vi "DataFileCreator2.vi"(10 "ProjectName":string="PrWave", 11 "Folder path input":path=path "C:/Users/Lab/Desktop/Data/DataBristol") -> (2 "NewFileCreated":string, 3 "NewFilePath":path)   [LabVIEW 2016]
doc: "Given an input Folder path this VI creates the next data file in the format \n2017-09-17ProjectName#001\nIt only checks the latest file in the folder to decide if a sequence with today's date already exists.\nIf the file sequence has not been started, it creates one begining with #001\nIf it happens that it tries to create a file that already exists, a dialog pops up\nasking for a new name."
panel:
  out "File time stamps sorted by time":timestamp[](array[timestamp])
  out "Files in Folder sorted by time":path[](array[path])
  out "FileTypeExists?":bool
  out "date string":string
  out "YearNow":string
  out "DayNow":string
  out "MonthNow":string
  out "DayParsed":string
  out "MonthParsed":string
  out "YearParsed":string
  out "newest existing file":string
  # "Given an input Folder path this VI creates the next data file in the format \n2017-09-17ProjectName#001\nIt only checks the latest file in the folder to decide if \na sequence with today's date already exists.\nIf the file sequence has not been started, it creates one begining with #001\nIf it happens that it tries to create a file that already exists, a dialog pops up\nasking for a new name."
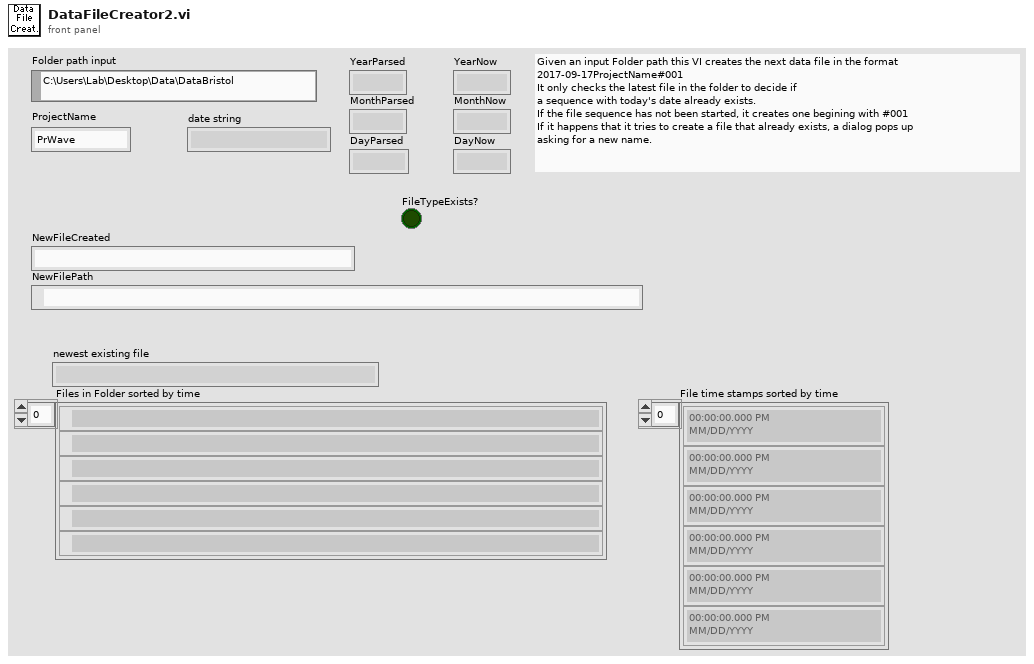
[diagram p1: front panel]
types:
  T1 = enum16{"open", "replace", "create", "open or create", "replace or create", "replace or create with confirmation"}
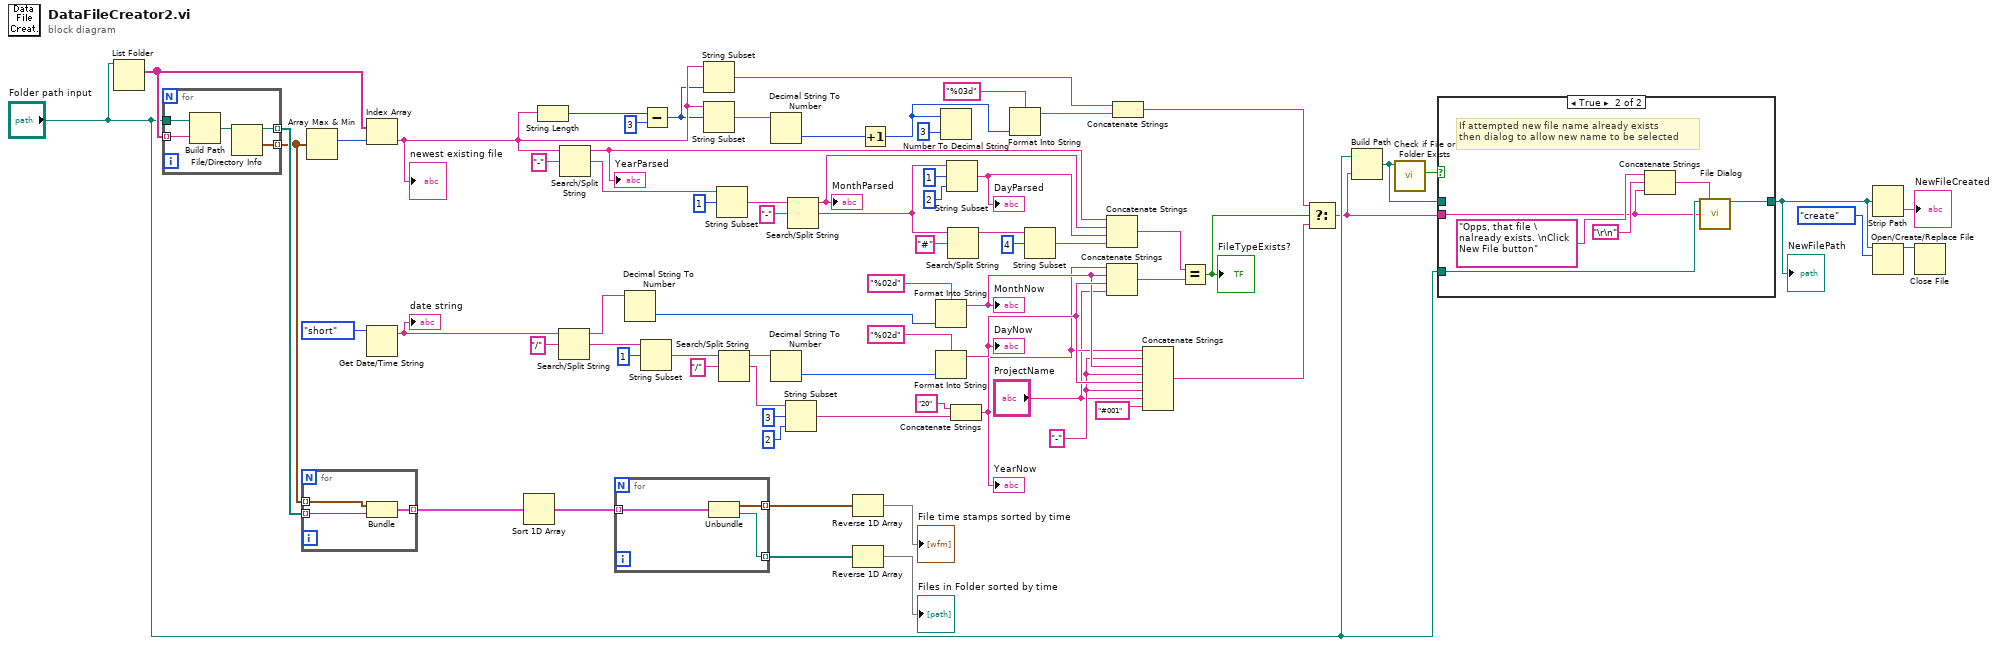
[diagram p0: block diagram]
diagram:
  w37 = "-" ("string")
  n1 = List Folder(path="Folder path input") -> (filenames=w51:string[])  [unwired: 3 in, 3 out]
  n2 = for {
    tunnel: w51 -> [w78] mode=indexing
    tunnel: [w76] -> w8 mode=indexing
    tunnel: [w75] -> w7 mode=indexing
    tunnel: "Folder path input" -> [w74]
    n3 = Build Path(base path=w74, name or relative path=w78) -> (appended path=w77:path)
    n4 = File/Directory Info(path=w77) -> (path out=w76:path, last mod=w75:timestamp)  [unwired: 1 in, 5 out]
  }
  n5 = for {
    tunnel: w7 -> [w81] mode=indexing
    tunnel: w8 -> [w80] mode=indexing
    tunnel: [w79] -> w14 mode=indexing
    n6 = Bundle("last mod"=w81, "path out"=w80) -> (w79:cluster{"last mod":timestamp, "path out":path})  [unwired: 1 in]
  }
  n7 = Array Max & Min(array=w7) -> (max index (indices)=w52:i32)  [unwired: 3 out]
  n8 = Index Array(array=w51, index=w52) -> (element=w42:string)
  "newest existing file" <- w42
  n9 = Get Date/Time String(date format (0)=enum16{"short", "long", "abbreviated"}."short") -> (date string=w55:string)  [unwired: 2 in, 1 out]
  "date string" <- w55
  n10 = Sort 1D Array(array=w14) -> (sorted array=w13:cluster{"last mod":timestamp, "path out":path}[])
  n11 = String Length(string=w42) -> (length=w32:i32)
  n12 = Search/Split String(string=w55, search string/char (-)="/") -> (substring before match=w47:string, match + rest of string=w63:string)  [unwired: 1 in, 1 out]
  n13 = Search/Split String(string=w42, search string/char (-)="-") -> (substring before match=w41:string, match + rest of string=w70:string)  [unwired: 1 in, 1 out]
  "YearParsed" <- w41
  n14 = for {
    tunnel: w13 -> [w84] mode=indexing
    tunnel: [w83] -> w11 mode=indexing
    tunnel: [w82] -> w12 mode=indexing
    n15 = Unbundle(w84) -> ("last mod"=w82:timestamp, "path out"=w83:path)
  }
  n16 = Decimal String To Number(string=w47) -> (number=w46:i32)  [unwired: 2 in, 1 out]
  n17 = String Subset(string=w63, offset (0)=1) -> (substring=w62:string)  [unwired: 1 in]
  n18 = Subtract(x=w32, y=3) -> (x-y=w30:i32)
  n19 = String Subset(string=w42, length (rest)=w30) -> (substring=w24:string)  [unwired: 1 in]
  n20 = String Subset(string=w42, offset (0)=w30) -> (substring=w29:string)  [unwired: 1 in]
  n21 = String Subset(string=w70, offset (0)=1) -> (substring=w69:string)  [unwired: 1 in]
  n22 = Search/Split String(string=w62, search string/char (-)="/") -> (substring before match=w43:string, match + rest of string=w60:string)  [unwired: 1 in, 1 out]
  n23 = Decimal String To Number(string=w29) -> (number=w28:i32)  [unwired: 2 in, 1 out]
  n24 = Decimal String To Number(string=w43) -> (number=w44:i32)  [unwired: 2 in, 1 out]
  n25 = String Subset(string=w60, offset (0)=3, length (rest)=2 ("y")) -> (substring=w57:string)
  n26 = Search/Split String(string=w69, search string/char (-)="-") -> (substring before match=w54:string, match + rest of string=w4:string)  [unwired: 1 in, 1 out]
  "MonthParsed" <- w54
  n27 = Reverse 1D Array(array=w12) -> (reversed array=→"File time stamps sorted by time":timestamp[])
  n28 = Reverse 1D Array(array=w11) -> (reversed array=→"Files in Folder sorted by time":path[])
  n29 = Increment(x=w28) -> (x+1=w26:i32)
  n30 = Format Into String(format string="%02d", w46) -> (resulting string=w39:string)  [unwired: 2 in, 1 out]
  "MonthNow" <- w39
  n31 = Format Into String(format string="%02d", w44) -> (resulting string=w40:string)  [unwired: 2 in, 1 out]
  "DayNow" <- w40
  n32 = Number To Decimal String(number=w26, width (-)=i16 3) -> ()  [unwired: 1 out]
  n33 = String Subset(string=w4, offset (0)=1, length (rest)=2 ("y")) -> (substring=w53:string)
  "DayParsed" <- w53
  n34 = Search/Split String(string=w4, search string/char (-)="#") -> (substring before match=w3:string)  [unwired: 1 in, 2 out]
  n35 = Concatenate Strings("20" ("string"), w57) -> (w38:string)
  "YearNow" <- w38
  n36 = Format Into String(format string="%03d", w26) -> (resulting string=w23:string)  [unwired: 2 in, 1 out]
  n37 = String Subset(string=w3, offset (0)=4) -> (substring=w2:string)  [unwired: 1 in]
  n38 = Concatenate Strings(w41, w54, w53, w2) -> (w50:string)
  n39 = Concatenate Strings(w38, w39, w40, "ProjectName") -> (w49:string)
  n40 = Concatenate Strings(w24, w23) -> (w34:string)
  n41 = Concatenate Strings(w38, w37, w39, w37, w40, w37, "ProjectName", "#001" ("string")) -> (w33:string)
  n42 = Equal?(x=w50, y=w49) -> (x = y?=w35:bool)
  "FileTypeExists?" <- w35
  n43 = Select(t=w34, s=w35, f=w33) -> (s? t:f=w17:string)
  n44 = Build Path(base path="Folder path input", name or relative path=w17) -> (appended path=w22:path)
  n45 = call <vilib>:"Check if File or Folder Exists.vi"("path"=w22) -> ("file or folder exists?"=w21:bool)  [unwired: 8 in, 2 out]
  n46 = case shown="True" w21 {
    tunnel: w22 -> [w85 _]
    tunnel: "Folder path input" -> [_ w91]
    tunnel: [w85 w90] -> w15
    tunnel: w17 -> [_ w86]
    frame False {
      # "If attempted name does not exist then \ncreate it"
    }
    frame True {
      # "If attempted new file name already exists\nthen dialog to allow new name to be selected"
      n47 = Concatenate Strings("Opps, that file \nalready exists. \nClick New File button" ("prompt"), "\r\n", w86) -> (w87:string)
      n48 = call "File Dialog"("start path"=w91, "prompt"=w87, "default name"=w86) -> ("selected path"=w90:path)  [unwired: 9 in, 3 out]
    }
  }
  "NewFilePath" <- w15
  n49 = Strip Path(path=w15) -> (name=→"NewFileCreated":string)  [unwired: 1 out]
  n50 = Open/Create/Replace File(file path (use dialog)=w15, operation (0:open)=T1."create") -> (refnum out=w18:refnum<file>)  [unwired: 4 in, 2 out]
  n51 = Close File(refnum=w18) -> ()  [unwired: 1 in, 2 out]
